vi "Range Kontrol Y.vi"(0 "denge degeri":dbl, 1 "iterasyon Denge":dbl=1.0, 2 "frekans index":dbl, 3 "Denge Kosulu y1_y2":dbl[][](array[numeric]), 4 "Yk":dbl, 5 "Y(k-1)":dbl=0.1, 6 "output y 1":dbl, 7 "output y 2":dbl) -> (14 "Output Y(k-1)":dbl=0.1, 15 "result output y":dbl, 18 "KONTROL X":bool, 19 "IF ELSE":bool)   [LabVIEW 2014]
uses:
  Sub_VI/show_sensitivity.vi
  Sub_VI/global get findinput.vi
panel:
  in  "GPIB In":refnum<visa-resource-name>="GPIB0::8::INSTR"
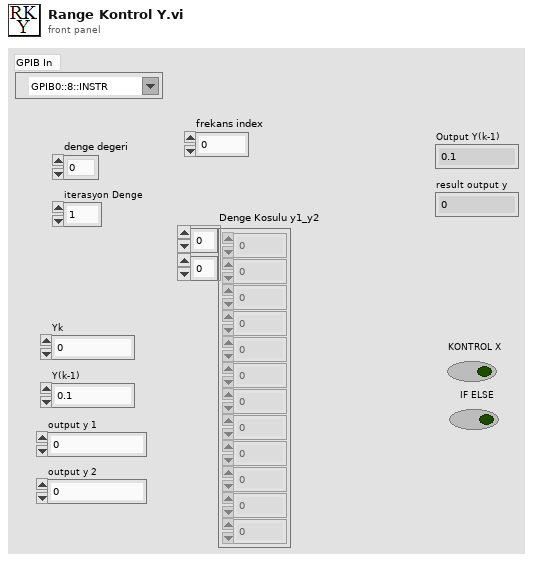
[diagram p1: front panel]
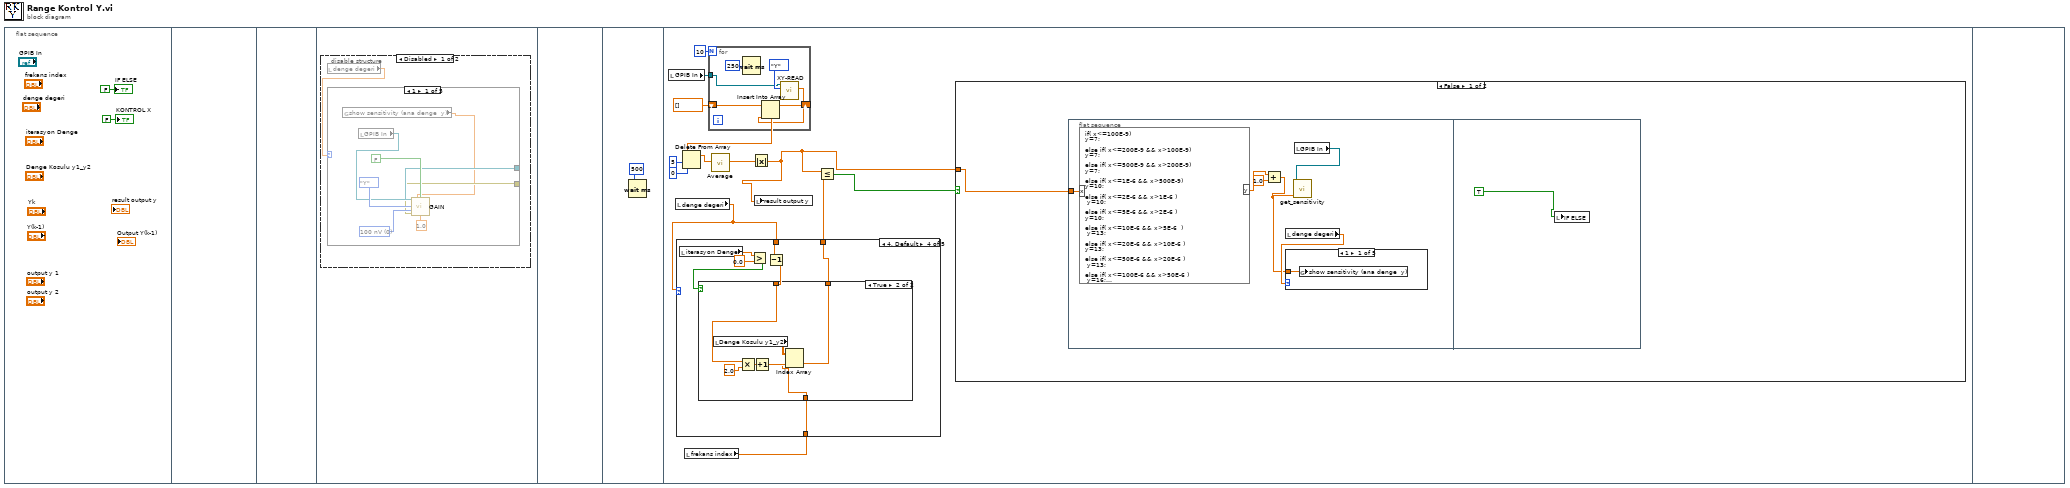
[diagram p0: block diagram]
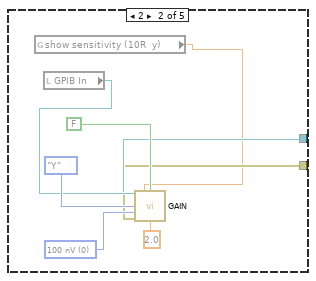
[diagram p2: hidden frame]
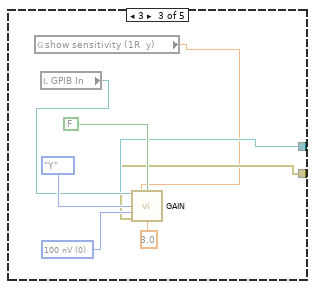
[diagram p3: hidden frame]
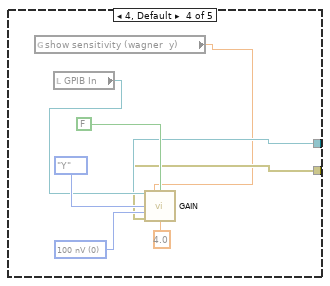
[diagram p4: hidden frame]
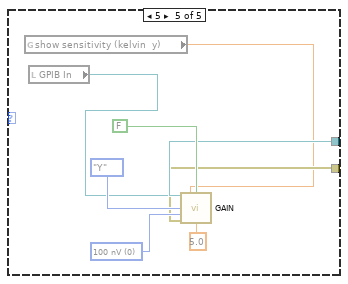
[diagram p5: hidden frame]
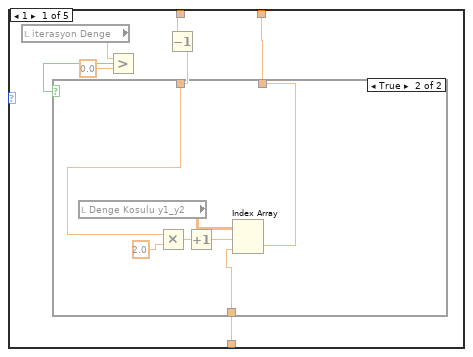
[diagram p7: hidden frame]
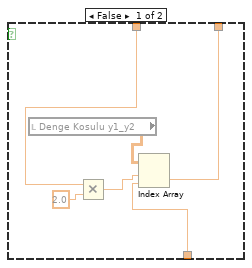
[diagram p8: hidden frame]
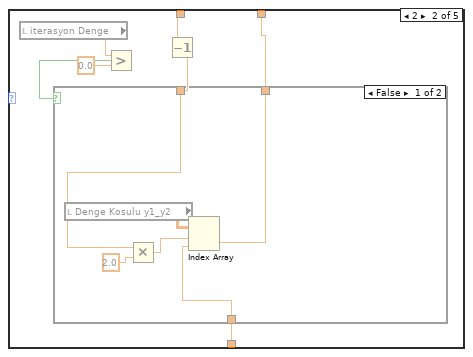
[diagram p9: hidden frame]
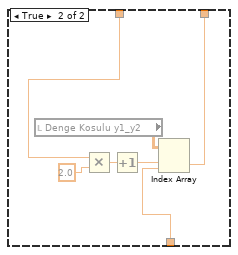
[diagram p10: hidden frame]
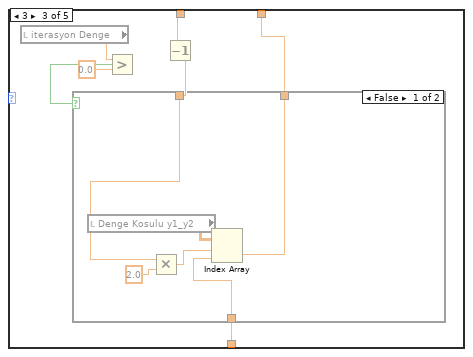
[diagram p11: hidden frame]
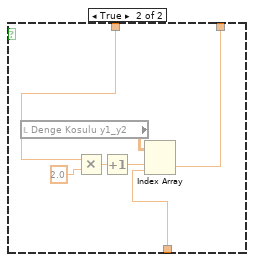
[diagram p12: hidden frame]
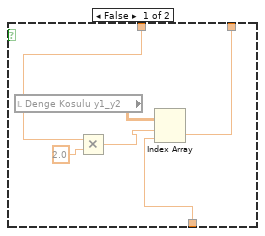
[diagram p13: hidden frame]
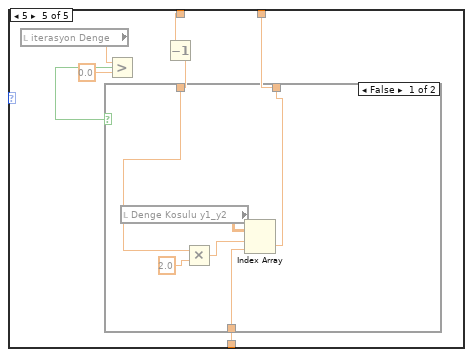
[diagram p14: hidden frame]
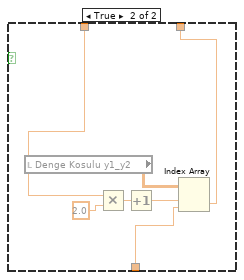
[diagram p15: hidden frame]
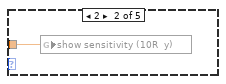
[diagram p16: hidden frame]
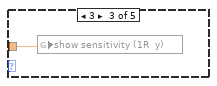
[diagram p17: hidden frame]
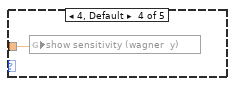
[diagram p18: hidden frame]
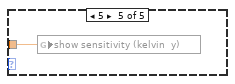
[diagram p19: hidden frame]
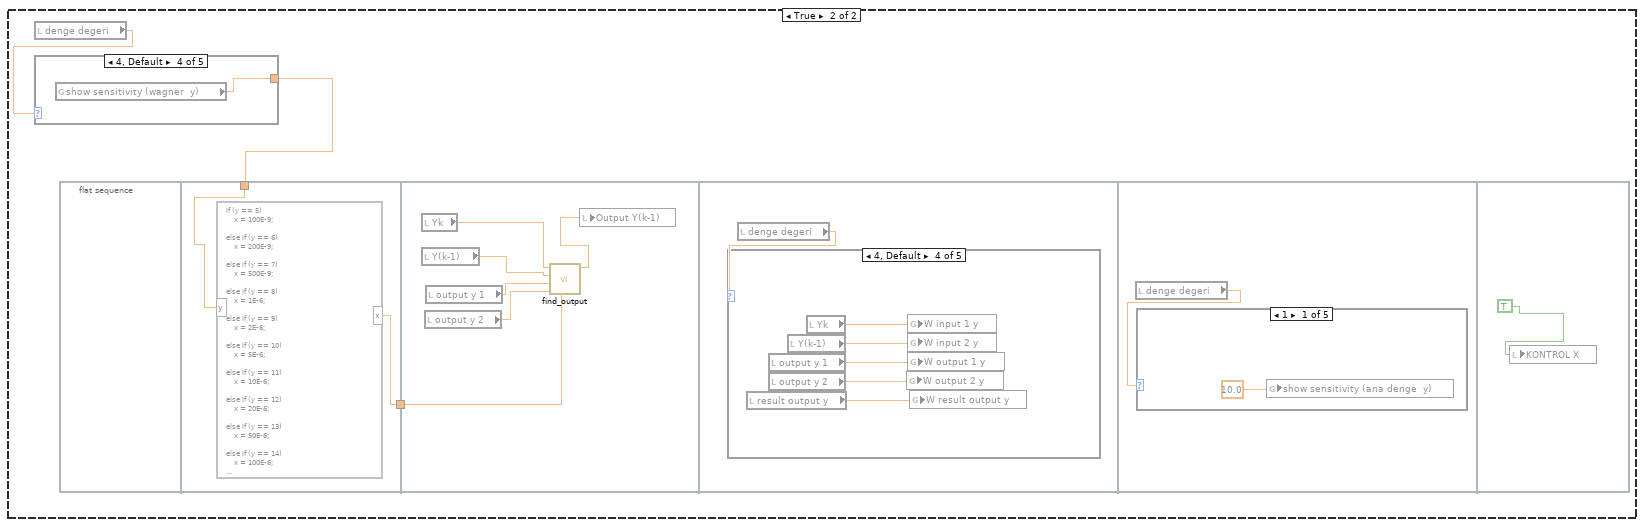
[diagram p20: hidden frame]
diagram:
  n1 = flat-sequence {
    frame #0 {
      "IF ELSE" <- FALSE ("IF ELSE")
      "KONTROL X" <- FALSE ("KONTROL X")
    }
    frame #1 {
    }
    frame #2 {
    }
    frame #3 {
      n2 = disable-structure shown="Disabled" {
        frame Disabled {
          n3 = local read "denge degeri"() -> (w5:dbl)
          n4 = case shown="1" w5 {
            tunnel: [w8 w16 w24 w32 w41] -> w4
            tunnel: [w7 w15 w23 w31 w40] -> w3
            frame 1 {
              w10 = u16 0 items=["100 nV", "200 nV", "500 nV", "1 uV", "2 uV", "5 uV", "10 uV", "20 uV", "50 uV", "100 uV", "200 uV", "500 uV", "1 mV"] ("Min. Hassasiyet")
              n5 = global read "show_sensitivity.vi" "show sensitivity (ana denge  y)"() -> (w6:dbl)
              n6 = local read "GPIB In"() -> (w11:refnum<visa-resource-name>)
              n7 = call "GAIN.vi"("SR850 GPIB In"=w11, "Max. Hassasiyet"=w6, "Auto Gain (False)"=FALSE, "Enum"=enum16{"X", "Y"}."Y", "Min. Hassasiyet"=w10, "choose"=1.0) -> ("SR850 GPIB Out"=w8:refnum<visa-resource-name>, "error out"=w7:errorcluster)  [unwired: 7 in, 1 out]
            }
            frame 2 {
              w18 = u16 0 items=["100 nV", "200 nV", "500 nV", "1 uV", "2 uV", "5 uV", "10 uV", "20 uV", "50 uV", "100 uV", "200 uV", "500 uV", "1 mV"] ("Min. Hassasiyet")
              n8 = global read "show_sensitivity.vi" "show sensitivity (10R  y)"() -> (w14:dbl)
              n9 = local read "GPIB In"() -> (w19:refnum<visa-resource-name>)
              n10 = call "GAIN.vi"("SR850 GPIB In"=w19, "Max. Hassasiyet"=w14, "Auto Gain (False)"=FALSE, "Enum"=enum16{"X", "Y"}."Y", "Min. Hassasiyet"=w18, "choose"=2.0) -> ("SR850 GPIB Out"=w16:refnum<visa-resource-name>, "error out"=w15:errorcluster)  [unwired: 7 in, 1 out]
            }
            frame 3 {
              w26 = u16 0 items=["100 nV", "200 nV", "500 nV", "1 uV", "2 uV", "5 uV", "10 uV", "20 uV", "50 uV", "100 uV", "200 uV", "500 uV", "1 mV"] ("Min. Hassasiyet")
              n11 = global read "show_sensitivity.vi" "show sensitivity (1R  y)"() -> (w22:dbl)
              n12 = local read "GPIB In"() -> (w27:refnum<visa-resource-name>)
              n13 = call "GAIN.vi"("SR850 GPIB In"=w27, "Max. Hassasiyet"=w22, "Auto Gain (False)"=FALSE, "Enum"=enum16{"X", "Y"}."Y", "Min. Hassasiyet"=w26, "choose"=3.0) -> ("SR850 GPIB Out"=w24:refnum<visa-resource-name>, "error out"=w23:errorcluster)  [unwired: 7 in, 1 out]
            }
            frame 4, Default {
              w34 = u16 0 items=["100 nV", "200 nV", "500 nV", "1 uV", "2 uV", "5 uV", "10 uV", "20 uV", "50 uV", "100 uV", "200 uV", "500 uV", "1 mV"] ("Min. Hassasiyet")
              n14 = global read "show_sensitivity.vi" "show sensitivity (wagner  y)"() -> (w30:dbl)
              n15 = local read "GPIB In"() -> (w35:refnum<visa-resource-name>)
              n16 = call "GAIN.vi"("SR850 GPIB In"=w35, "Max. Hassasiyet"=w30, "Auto Gain (False)"=FALSE, "Enum"=enum16{"X", "Y"}."Y", "Min. Hassasiyet"=w34, "choose"=4.0) -> ("SR850 GPIB Out"=w32:refnum<visa-resource-name>, "error out"=w31:errorcluster)  [unwired: 7 in, 1 out]
            }
            frame 5 {
              w43 = u16 0 items=["100 nV", "200 nV", "500 nV", "1 uV", "2 uV", "5 uV", "10 uV", "20 uV", "50 uV", "100 uV", "200 uV", "500 uV", "1 mV"] ("Min. Hassasiyet")
              n17 = global read "show_sensitivity.vi" "show sensitivity (kelvin  y)"() -> (w39:dbl)
              n18 = local read "GPIB In"() -> (w38:refnum<visa-resource-name>)
              n19 = call "GAIN.vi"("SR850 GPIB In"=w38, "Max. Hassasiyet"=w39, "Auto Gain (False)"=FALSE, "Enum"=enum16{"X", "Y"}."Y", "Min. Hassasiyet"=w43, "choose"=5.0) -> ("SR850 GPIB Out"=w41:refnum<visa-resource-name>, "error out"=w40:errorcluster)  [unwired: 7 in, 1 out]
            }
          }
        }
        frame Enabled {
        }
      }
    }
    frame #4 {
    }
    frame #5 {
      n20 = Wait (ms)(milliseconds to wait=u32 500) -> ()  [unwired: 1 out]
    }
    frame #6 {
      n21 = local read "GPIB In"() -> (w47:refnum<visa-resource-name>)
      n22 = local read "denge degeri"() -> (w50:dbl)
      n23 = local read "frekans index"() -> (w48:dbl)
      n24 = case shown="4, Default" w50 {
        tunnel: [w63 w83 w103 w126 w143] -> w51
        tunnel: w50 -> [w62 w82 w102 w122 w142]
        tunnel: w48 -> [w60 w80 w100 w120 w140]
        frame 1 {
          n25 = local read "iterasyon Denge"() -> (w65:dbl)
          n26 = Greater?(x=w65, y=0.0) -> (0:w66:bool)
          n27 = Decrement(x=w62) -> (x-1=w61:dbl)
          n28 = case shown="True" w66 {
            tunnel: [w70 w76] -> w63
            tunnel: w61 -> [w69 w75]
            tunnel: w60 -> [w67 w73]
            frame False {
              n29 = local read "Denge Kosulu y1_y2"() -> (w72:dbl[][])
              n30 = Multiply(x=w69, y=2.0) -> (x*y=w68:dbl)
              n31 = Index Array(array=w72, index (row)=w68, index (col)=w67) -> (element=w70:dbl)
            }
            frame True {
              n32 = local read "Denge Kosulu y1_y2"() -> (w77:dbl[][])
              n33 = Multiply(x=w75, y=2.0) -> (x*y=w79:dbl)
              n34 = Increment(x=w79) -> (x+1=w74:dbl)
              n35 = Index Array(array=w77, index (row)=w74, index (col)=w73) -> (element=w76:dbl)
            }
          }
        }
        frame 2 {
          n36 = local read "iterasyon Denge"() -> (w85:dbl)
          n37 = Greater?(x=w85, y=0.0) -> (0:w86:bool)
          n38 = Decrement(x=w82) -> (x-1=w81:dbl)
          n39 = case shown="False" w86 {
            tunnel: [w90 w96] -> w83
            tunnel: w81 -> [w89 w95]
            tunnel: w80 -> [w87 w93]
            frame False {
              n40 = local read "Denge Kosulu y1_y2"() -> (w92:dbl[][])
              n41 = Multiply(x=w89, y=2.0) -> (x*y=w88:dbl)
              n42 = Index Array(array=w92, index (row)=w88, index (col)=w87) -> (element=w90:dbl)
            }
            frame True {
              n43 = local read "Denge Kosulu y1_y2"() -> (w97:dbl[][])
              n44 = Multiply(x=w95, y=2.0) -> (x*y=w99:dbl)
              n45 = Increment(x=w99) -> (x+1=w94:dbl)
              n46 = Index Array(array=w97, index (row)=w94, index (col)=w93) -> (element=w96:dbl)
            }
          }
        }
        frame 3 {
          n47 = local read "iterasyon Denge"() -> (w104:dbl)
          n48 = Greater?(x=w104, y=0.0) -> (0:w106:bool)
          n49 = Decrement(x=w102) -> (x-1=w101:dbl)
          n50 = case shown="False" w106 {
            tunnel: [w110 w116] -> w103
            tunnel: w101 -> [w109 w115]
            tunnel: w100 -> [w107 w113]
            frame False {
              n51 = local read "Denge Kosulu y1_y2"() -> (w112:dbl[][])
              n52 = Multiply(x=w109, y=2.0) -> (x*y=w108:dbl)
              n53 = Index Array(array=w112, index (row)=w108, index (col)=w107) -> (element=w110:dbl)
            }
            frame True {
              n54 = local read "Denge Kosulu y1_y2"() -> (w117:dbl[][])
              n55 = Multiply(x=w115, y=2.0) -> (x*y=w119:dbl)
              n56 = Increment(x=w119) -> (x+1=w114:dbl)
              n57 = Index Array(array=w117, index (row)=w114, index (col)=w113) -> (element=w116:dbl)
            }
          }
        }
        frame 4, Default {
          n58 = local read "iterasyon Denge"() -> (w124:dbl)
          n59 = Greater?(x=w124, y=0.0) -> (0:w123:bool)
          n60 = Decrement(x=w122) -> (x-1=w121:dbl)
          n61 = case shown="True" w123 {
            tunnel: [w130 w136] -> w126
            tunnel: w121 -> [w129 w135]
            tunnel: w120 -> [w127 w133]
            frame False {
              n62 = local read "Denge Kosulu y1_y2"() -> (w132:dbl[][])
              n63 = Multiply(x=w129, y=2.0) -> (x*y=w128:dbl)
              n64 = Index Array(array=w132, index (row)=w128, index (col)=w127) -> (element=w130:dbl)
            }
            frame True {
              n65 = local read "Denge Kosulu y1_y2"() -> (w137:dbl[][])
              n66 = Multiply(x=w135, y=2.0) -> (x*y=w139:dbl)
              n67 = Increment(x=w139) -> (x+1=w134:dbl)
              n68 = Index Array(array=w137, index (row)=w134, index (col)=w133) -> (element=w136:dbl)
            }
          }
        }
        frame 5 {
          n69 = local read "iterasyon Denge"() -> (w144:dbl)
          n70 = Greater?(x=w144, y=0.0) -> (0:w146:bool)
          n71 = Decrement(x=w142) -> (x-1=w141:dbl)
          n72 = case shown="False" w146 {
            tunnel: [w150 w156] -> w143
            tunnel: w141 -> [w149 w155]
            tunnel: w140 -> [w147 w153]
            frame False {
              n73 = local read "Denge Kosulu y1_y2"() -> (w152:dbl[][])
              n74 = Multiply(x=w149, y=2.0) -> (x*y=w148:dbl)
              n75 = Index Array(array=w152, index (row)=w148, index (col)=w147) -> (element=w150:dbl)
            }
            frame True {
              n76 = local read "Denge Kosulu y1_y2"() -> (w157:dbl[][])
              n77 = Multiply(x=w155, y=2.0) -> (x*y=w159:dbl)
              n78 = Increment(x=w159) -> (x+1=w154:dbl)
              n79 = Index Array(array=w157, index (row)=w154, index (col)=w153) -> (element=w156:dbl)
            }
          }
        }
      }
      n80 = for {
        N: 10 -> [_]
        shift-right: [w224] -> w56
        shift-left: dbl[] [] -> [w225]
        tunnel: w47 -> [w222]
        n81 = Wait (ms)(milliseconds to wait=u32 250) -> ()  [unwired: 1 out]
        n82 = call "XY-READ.vi"("X/Y ?"=enum16{"X", "Y"}."Y" ("Enum"), "SR850 GPIB IN"=w222) -> ("SR850_Reading"=w226:dbl)  [unwired: 7 in, 2 out]
        n83 = Insert Into Array(array=w225, new element=w226) -> (w224:dbl[])  [unwired: 1 in]
      }
      n84 = Delete From Array(array=w56, length=5, index=0) -> (array with subset deleted=w57:dbl[])  [unwired: 1 out]
      n85 = call "Average.vi"("Array"=w57) -> ("Average"=w53:dbl)  [unwired: 9 in, 1 out]
      n86 = Absolute Value(x=w53) -> (abs(x)=w49:dbl)
      n87 = local write "result output y"(w49) -> ()
      n88 = Less Or Equal?(x=w49, y=w51) -> (x <= y?=w52:bool)
      n89 = case shown="False" w52 {
        tunnel: w49 -> [w160 _]
        frame False {
          n90 = flat-sequence {
            tunnel: w160 -> [w165]
            frame #0 {
              n91 = formula code="if( x<=100E-9) \ny=7;\n\nelse if( x<=200E-9 && x>100E-9) \ny=7;\n\nelse if( x<=500E-9 && x>200E-9) \ny=7;\n\nelse if( x<=1E-6 && x>500E-9) \ny=10;\n\nelse if( x<=2E-6 && x>1E-6 ) \n\ty=10;\n\nelse if( x<=5E-6 && x>2E-6 ) \ny=10;\n\nelse if( x<=10E-6 && x>5E-6  ) \n\ty=13;\n\nelse if( x<=20E-6 && x>10E-6 ) \ny=13;\n\nelse if( x<=50E-6 && x>20E-6 ) \n\ty=13;\n\nelse if( x<=100E-6 && x>50E-6 ) \n\ty=16;\n\nelse if( x<=200E-6 && x>100E-6 ) \n\ty=16;\n\nelse if( x<=500E-6 && x>200E-6 ) \n\ty=16;\n\nelse if(  x<=1E-3 && x>500E-6 ) \n\ty=19;\n\nelse if( x<=2E-3 && x>1E-3 ) \n\ty=19;\n\nelse if(  x<=5E-3 && x>2E-3) \ny=19;\n\nelse if(  x<=10E-3 && x>5E-3 ) \n\ty=22;\n\nelse if(  x<=20E-3 && x>10E-3) \n\ty=22;\n\nelse if(  x<=50E-3 && x>20E-3 ) \n\ty=22;\n\nelse if(  x<=100E-3 && x>50E-3 ) \n\ty=25;\n\nelse if(  x<=200E-3 && x>100E-3 ) \n\ty=25;\n\nelse if(  x<=500E-3 && x>200E-3 ) \n\ty=25;\n\nelse if(  x<=1 && x>500E-3 ) \ny=26;\n\nelse \n\ty=26;"("x"=w165) -> ("y"=w163:dbl)
              n92 = Add(x=w163, y=1.0) -> (x+y=w161:dbl)
              n93 = local read "denge degeri"() -> (w164:dbl)
              n94 = case shown="1" w164 {
                tunnel: w161 -> [w167 w168 w169 w170 w171]
                frame 1 {
                  n95 = global write "show_sensitivity.vi" "show sensitivity (ana denge  y)"(w167) -> ()
                }
                frame 2 {
                  n96 = global write "show_sensitivity.vi" "show sensitivity (10R  y)"(w168) -> ()
                }
                frame 3 {
                  n97 = global write "show_sensitivity.vi" "show sensitivity (1R  y)"(w169) -> ()
                }
                frame 4, Default {
                  n98 = global write "show_sensitivity.vi" "show sensitivity (wagner  y)"(w170) -> ()
                }
                frame 5 {
                  n99 = global write "show_sensitivity.vi" "show sensitivity (kelvin  y)"(w171) -> ()
                }
              }
              n100 = local read "GPIB In"() -> (w166:refnum<visa-resource-name>)
              n101 = call "get_sensitivity.vi"("input 1"=w161, "SR850 GPIB In"=w166) -> ()  [unwired: 8 in, 2 out]
            }
            frame #1 {
              n102 = local write "IF ELSE"(TRUE ("if else")) -> ()
            }
          }
        }
        frame True {
          n103 = local read "denge degeri"() -> (w175:dbl)
          n104 = case shown="4, Default" w175 {
            tunnel: [w217 w218 w219 w220 w221] -> w173
            frame 1 {
              n105 = global read "show_sensitivity.vi" "show sensitivity (ana denge  y)"() -> (w217:dbl)
            }
            frame 2 {
              n106 = global read "show_sensitivity.vi" "show sensitivity (10R  y)"() -> (w218:dbl)
            }
            frame 3 {
              n107 = global read "show_sensitivity.vi" "show sensitivity (1R  y)"() -> (w219:dbl)
            }
            frame 4, Default {
              n108 = global read "show_sensitivity.vi" "show sensitivity (wagner  y)"() -> (w220:dbl)
            }
            frame 5 {
              n109 = global read "show_sensitivity.vi" "show sensitivity (kelvin  y)"() -> (w221:dbl)
            }
          }
          n110 = flat-sequence {
            tunnel: w173 -> [w176]
            tunnel: [w177] -> w174
            tunnel: w174 -> [w181]
            frame #0 {
            }
            frame #1 {
              n111 = formula code="if (y == 5) \n    x = 100E-9;\n\nelse if (y == 6) \n    x = 200E-9;\n\nelse if (y == 7) \n    x = 500E-9;\n\nelse if (y == 8) \n    x = 1E-6;\n\nelse if (y == 9) \n    x = 2E-6;\n\nelse if (y == 10) \n    x = 5E-6;\n\nelse if (y == 11) \n    x = 10E-6;\n\nelse if (y == 12) \n    x = 20E-6;\n\nelse if (y == 13) \n    x = 50E-6;\n\nelse if (y == 14) \n    x = 100E-6;\n\nelse if (y == 15) \n    x = 200E-6;\n\nelse if (y == 16) \n    x = 500E-6;\n\nelse if (y == 17) \n    x = 1E-3;\n\nelse if (y == 18) \n    x = 2E-3;\n\nelse if (y == 19) \n    x = 5E-3;\n\nelse if (y == 20) \n    x = 10E-3;\n\nelse if (y == 21) \n    x = 20E-3;\n\nelse if (y == 22) \n    x = 50E-3;\n\nelse if (y == 23) \n    x = 100E-3;\n\nelse if (y == 24) \n    x = 200E-3;\n\nelse if (y == 25) \n    x = 500E-3;\n\nelse if (y == 26) \n    x = 1;\n\nelse \n    x = 1;"("y"=w176) -> ("x"=w177:dbl)
            }
            frame #2 {
              n112 = local read "Yk"() -> (w179:dbl)
              n113 = local read "Y(k-1)"() -> (w180:dbl)
              n114 = local read "output y 2"() -> (w182:dbl)
              n115 = local read "output y 1"() -> (w183:dbl)
              n116 = call "find_output.vi"("find output"=w181, "output 2"=w182, "output 1"=w183, "input 2"=w180, "input 1"=w179) -> ("getInput"=w178:dbl)  [unwired: 6 in]
              n117 = local write "Output Y(k-1)"(w178) -> ()
            }
            frame #3 {
              n118 = local read "denge degeri"() -> (w184:dbl)
              n119 = case shown="4, Default" w184 {
                frame 1 {
                  n120 = local read "result output y"() -> (w185:dbl)
                  n121 = local read "output y 1"() -> (w187:dbl)
                  n122 = local read "output y 2"() -> (w186:dbl)
                  n123 = local read "Y(k-1)"() -> (w188:dbl)
                  n124 = local read "Yk"() -> (w189:dbl)
                  n125 = global write "global get findinput.vi" "AD input 1 y"(w189) -> ()
                  n126 = global write "global get findinput.vi" "AD input 2 y"(w188) -> ()
                  n127 = global write "global get findinput.vi" "AD output 1 y"(w187) -> ()
                  n128 = global write "global get findinput.vi" "AD output 2 y"(w186) -> ()
                  n129 = global write "global get findinput.vi" "AD result output y"(w185) -> ()
                }
                frame 2 {
                  n130 = local read "result output y"() -> (w190:dbl)
                  n131 = local read "output y 1"() -> (w192:dbl)
                  n132 = local read "output y 2"() -> (w191:dbl)
                  n133 = local read "Y(k-1)"() -> (w193:dbl)
                  n134 = local read "Yk"() -> (w194:dbl)
                  n135 = global write "global get findinput.vi" "10R input 1 y"(w194) -> ()
                  n136 = global write "global get findinput.vi" "10R input 2 y"(w193) -> ()
                  n137 = global write "global get findinput.vi" "10R output 1 y"(w192) -> ()
                  n138 = global write "global get findinput.vi" "10R result output y"(w190) -> ()
                  n139 = global write "global get findinput.vi" "10R output 2 y"(w191) -> ()
                }
                frame 3 {
                  n140 = local read "result output y"() -> (w195:dbl)
                  n141 = local read "output y 1"() -> (w197:dbl)
                  n142 = local read "output y 2"() -> (w196:dbl)
                  n143 = local read "Y(k-1)"() -> (w198:dbl)
                  n144 = local read "Yk"() -> (w199:dbl)
                  n145 = global write "global get findinput.vi" "1R input 1 y"(w199) -> ()
                  n146 = global write "global get findinput.vi" "1R output 1 y"(w197) -> ()
                  n147 = global write "global get findinput.vi" "1R output 2 y"(w196) -> ()
                  n148 = global write "global get findinput.vi" "1R input 2 y"(w198) -> ()
                  n149 = global write "global get findinput.vi" "1R result output y"(w195) -> ()
                }
                frame 4, Default {
                  n150 = local read "result output y"() -> (w200:dbl)
                  n151 = local read "output y 1"() -> (w202:dbl)
                  n152 = local read "output y 2"() -> (w201:dbl)
                  n153 = local read "Y(k-1)"() -> (w203:dbl)
                  n154 = local read "Yk"() -> (w204:dbl)
                  n155 = global write "global get findinput.vi" "W output 2 y"(w201) -> ()
                  n156 = global write "global get findinput.vi" "W input 1 y"(w204) -> ()
                  n157 = global write "global get findinput.vi" "W input 2 y"(w203) -> ()
                  n158 = global write "global get findinput.vi" "W output 1 y"(w202) -> ()
                  n159 = global write "global get findinput.vi" "W result output y"(w200) -> ()
                }
                frame 5 {
                  n160 = local read "result output y"() -> (w205:dbl)
                  n161 = local read "output y 1"() -> (w207:dbl)
                  n162 = local read "output y 2"() -> (w206:dbl)
                  n163 = local read "Y(k-1)"() -> (w208:dbl)
                  n164 = local read "Yk"() -> (w209:dbl)
                  n165 = global write "global get findinput.vi" "KV result output y"(w205) -> ()
                  n166 = global write "global get findinput.vi" "KV input 2 y"(w208) -> ()
                  n167 = global write "global get findinput.vi" "KV input 1 y"(w209) -> ()
                  n168 = global write "global get findinput.vi" "KV output 1 y"(w207) -> ()
                  n169 = global write "global get findinput.vi" "KV output 2 y"(w206) -> ()
                }
              }
            }
            frame #4 {
              n170 = local read "denge degeri"() -> (w210:dbl)
              n171 = case shown="1" w210 {
                frame 1 {
                  n172 = global write "show_sensitivity.vi" "show sensitivity (ana denge  y)"(10.0 ("show sensitivity (kelvin  y)")) -> ()
                }
                frame 2 {
                  n173 = global write "show_sensitivity.vi" "show sensitivity (10R  y)"(16.0 ("show sensitivity (kelvin  y)")) -> ()
                }
                frame 3 {
                  n174 = global write "show_sensitivity.vi" "show sensitivity (1R  y)"(16.0 ("show sensitivity (kelvin  y)")) -> ()
                }
                frame 4, Default {
                  n175 = global write "show_sensitivity.vi" "show sensitivity (wagner  y)"(16.0 ("show sensitivity (kelvin  y)")) -> ()
                }
                frame 5 {
                  n176 = global write "show_sensitivity.vi" "show sensitivity (kelvin  y)"(10.0 ("show sensitivity (kelvin  y)")) -> ()
                }
              }
            }
            frame #5 {
              n177 = local write "KONTROL X"(TRUE ("KONTROL Y")) -> ()
            }
          }
        }
      }
    }
    frame #7 {
    }
  }
